vi "Calculate Velocity Setpoints.vi"() -> ()   [LabVIEW 2019]
panel:
  out "Right Setpoint":dbl
  out "Left Setpoint":dbl
  out "Wait Time (ms)":dbl
  out "Angles PID":cluster{"IPCed":dbl, "output 2":dbl}
  in  "PID gains":T1={"proportional gain (Kc)"=1.0, "integral time (Ti, min)"=0.01, "derivative time (Td, min)"=0.0} {"derivative time (Td, min)" format="%.3f"; "integral time (Ti, min)" format="%.3f"; "proportional gain (Kc)" format="%.3f"}
  in  "Angle To Get":dbl(slide) scale=0.0..360.0
  in  "Align?":bool
  in  "IMU Input":dbl
  in  "Enum":enum16{"JV", "Mule", "Linda/Sophie"}(ring)
  in  "Angular Data (Relative)":dbl[](array[numeric])
  in  "Velocity Data":dbl[](array[numeric])
  in  "Time":u32
  in  "Timestamp":i32
  in  "Front is Back":bool
  in  "Reversed":bool
  in  "Negated":bool
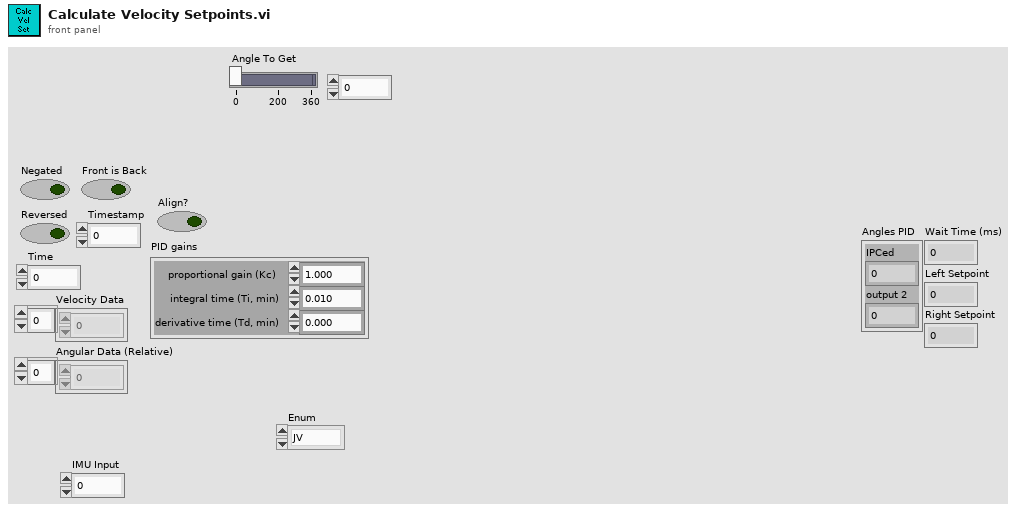
[diagram p1: front panel]
types:
  T1 = cluster{"proportional gain (Kc)":dbl, "integral time (Ti, min)":dbl, "derivative time (Td, min)":dbl}
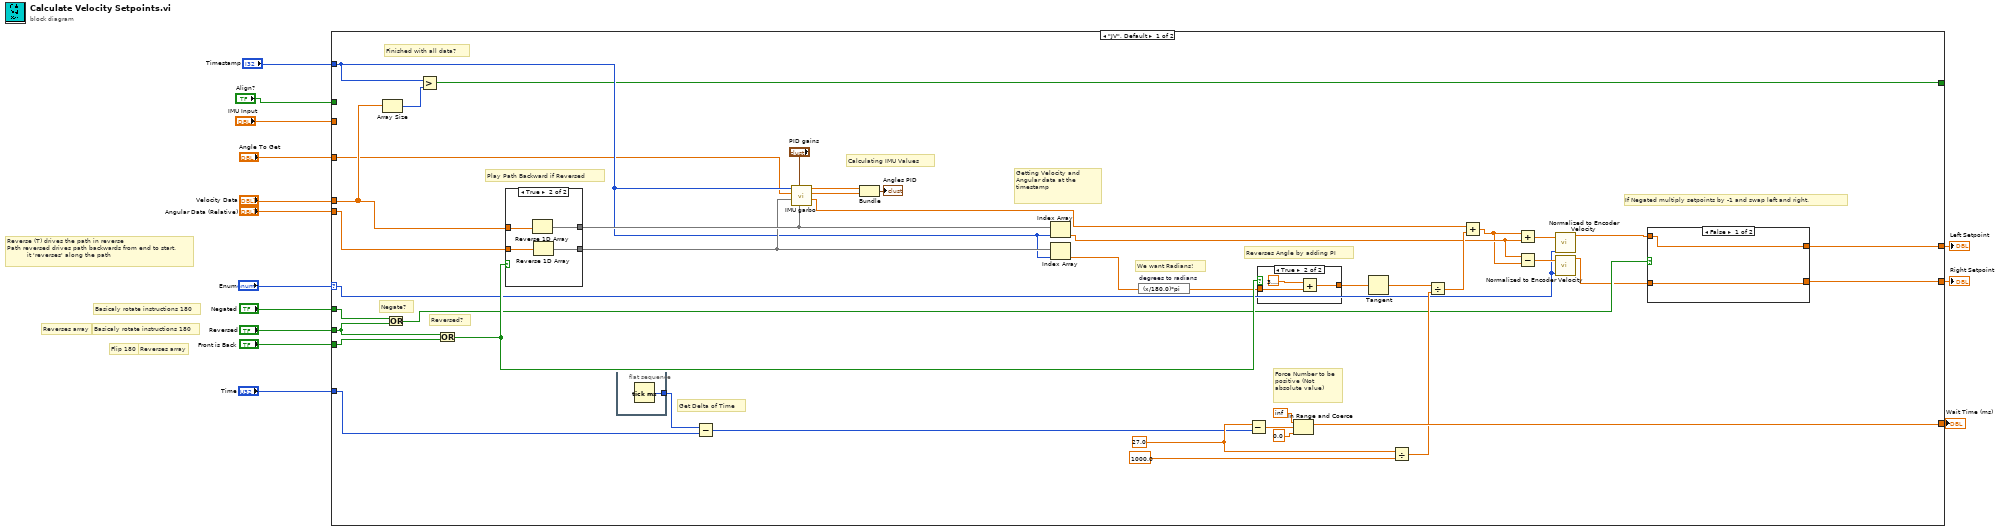
[diagram p0: block diagram]
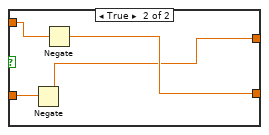
[diagram p2: hidden frame]
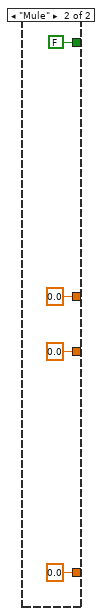
[diagram p5: hidden frame]
diagram:
  # "Reverse (T) drives the path in reverse\nPath reversed drives path backwards from end to start. \n          it 'reverses' along the path"
  # "Basicaly rotate instructions 180"
  # "Basicaly rotate instructions 180"
  # "Flip 180"
  # "Reverses array"
  # "Reverses array"
  n1 = case shown="\"JV\", Default" "Enum" {
    selector: "Enum" -> [w22 _]
    tunnel: "Negated" -> [w20 _]
    tunnel: "Reversed" -> [w21 _]
    tunnel: "Front is Back" -> [w56 _]
    tunnel: "Time" -> [w37 _]
    tunnel: "Angular Data (Relative)" -> [w55 _]
    tunnel: "Velocity Data" -> [w54 _]
    tunnel: "Angle To Get" -> [w48 _]
    tunnel: "IMU Input" -> [_ _]
    tunnel: "Align?" -> [_ _]
    tunnel: "Timestamp" -> [w49 _]
    tunnel: [w40 FALSE] -> _
    tunnel: [w31 0.0 ("lower limit")] -> w3
    tunnel: [w16 0.0 ("Output")] -> w2
    tunnel: [w15 0.0 ("Output")] -> w1
    frame "JV", Default {
      w38 = 27.0 ("x")
      # "If Negated multiply setpoints by -1 and swap left and right."
      # "Negate?"
      # "Force Number to be positive (Not absolute value)"
      # "Get Delta of Time"
      # "Finished with all data?"
      # "Reverses Angle by adding PI"
      # "We want Radians!"
      # "Calculating IMU Values"
      # "Getting Velocity and Angular data at the timestamp"
      # "Reversed?"
      # "Play Path Backward if Reversed"
      n2 = Array Size(array=w54) -> (size(s)=w53:i32)
      n3 = Or(x=w20, y=w21) -> (x .or. y?=w19:bool)
      n4 = Greater?(x=w49, y=w53) -> (0:w40:bool)
      n5 = Or(x=w21, y=w56) -> (x .or. y?=w43:bool)
      n6 = case shown="True" w43 {
        tunnel: w54 -> [w69 w73]
        tunnel: w55 -> [w68 w72]
        tunnel: [w69 w71] -> w52
        tunnel: [w68 w70] -> w51
        frame False {
        }
        frame True {
          n7 = Reverse 1D Array(array=w73) -> (reversed array=w71:dbl[])
          n8 = Reverse 1D Array(array=w72) -> (reversed array=w70:dbl[])
        }
      }
      n9 = flat-sequence {
        tunnel: [w63] -> w36
        frame #0 {
          n10 = Tick Count (ms)() -> (millisecond timer value=w63:u32)
        }
      }
      n11 = Subtract(x=w36, y=w37) -> (x-y=w35:u32)
      n12 = call "IMU garbo.vi"("Velocity Data"=w52, "PID gains"="PID gains", "Angular Data (Relative)"=w51, "Angle to Get"=w48, "Iterations"=w49) -> ("output"=w27:dbl, "output 2"=w46:dbl, "IPCed"=w47:dbl)  [unwired: 3 in, 1 out]
      n13 = Bundle("IPCed"=w47, "output 2"=w46) -> (→"Angles PID":cluster{"IPCed":dbl, "output 2":dbl})  [unwired: 1 in]
      n14 = Index Array(array=w52, index=w49) -> (element=w26:dbl)
      n15 = Index Array(array=w51, index=w49) -> (element=w44:dbl)
      n16 = expression code="(x/180.0)*pi" "degrees to radians"(w44) -> (w42:dbl)
      n17 = Subtract(x=w38, y=w35) -> (x-y=w34:dbl)
      n18 = case shown="True" w43 {
        tunnel: w42 -> [w64 w67]
        tunnel: [w64 w65] -> w41
        frame False {
        }
        frame True {
          n19 = Add(x=3.141592653589793, y=w67) -> (x+y=w65:dbl)
        }
      }
      n20 = In Range and Coerce(upper limit=inf, x=w34, lower limit=0.0) -> (coerced(x)=w31:dbl)  [unwired: 1 out]
      n21 = Tangent(1:w41) -> (0:w30:dbl)
      n22 = Divide(x=w38, y=1000.0) -> (x/y=w29:dbl)
      n23 = Divide(x=w30, y=w29) -> (x/y=w28:dbl)
      n24 = Add(x=w27, y=w28) -> (x+y=w25:dbl)
      n25 = Add(x=w25, y=w26) -> (x+y=w24:dbl)
      n26 = Subtract(x=w26, y=w25) -> (x-y=w23:dbl)
      n27 = call "Normalized to Encoder Velocity.vi"("Enum"=w22, "ft/s"=w24) -> ("Output"=w18:dbl)  [unwired: 9 in]
      n28 = call "Normalized to Encoder Velocity.vi"("Enum"=w22, "ft/s"=w23) -> ("Output"=w17:dbl)  [unwired: 9 in]
      n29 = case shown="False" w19 {
        tunnel: w18 -> [w58 w61]
        tunnel: w17 -> [w57 w62]
        tunnel: [w57 w60] -> w15
        tunnel: [w58 w59] -> w16
        frame False {
        }
        frame True {
          n30 = Negate(x=w62) -> (-x=w59:dbl)
          n31 = Negate(x=w61) -> (-x=w60:dbl)
        }
      }
    }
    frame "Mule" {
    }
  }
  "Wait Time (ms)" <- w3
  "Left Setpoint" <- w2
  "Right Setpoint" <- w1
